vi "LVClass_Camera Set CameraSet.vi"(0 "Camera in":refnum<class "Camera.lvclass">, 5 "CameraSet":refnum<class "CameraSet.lvclass">, 7 "load_and_apply_connection_params":bool, 9 "load_and_apply_params":bool, 11 "error in (no error)":errorcluster) -> (4 "Camera out":refnum<class "Camera.lvclass">, 15 "error out":errorcluster)   [LabVIEW 2020, in "Camera.lvclass"]
doc: "Load and apply camera parameters from a CameraSet object.\n\n<B>CameraIn</B> : Camera object.\n<B>CameraOut</B> : Camera object.\n<B>CameraSet</B> : CameraSet object.\n<B>load_and_apply_connection_params</B> : try to load and apply connection parameters if true\n<B>load_and_apply_params</B> : try to load and apply parameters if true."
uses:
  Camera.lvclass
  CameraSet.lvclass
  Camera.lvclass/Camera.ctl
  LVClass_CameraSet Read CameraSet.vi
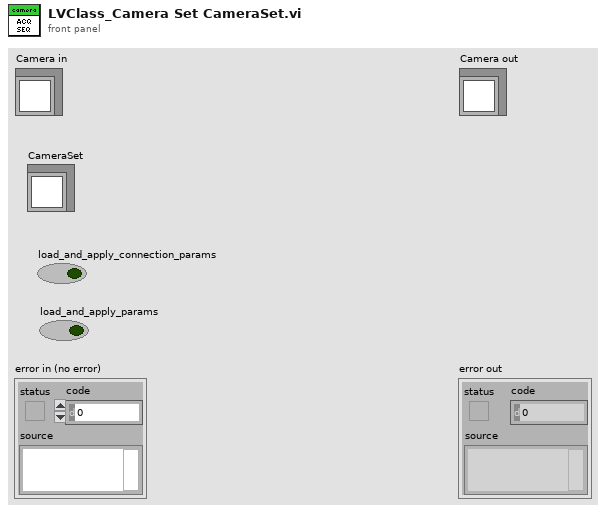
[diagram p1: front panel]
types:
  T1 = typedef "ClassID.ctl" = i64
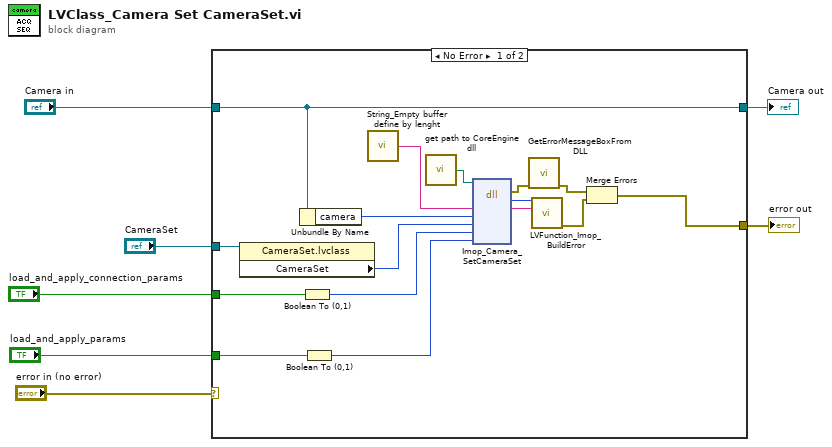
[diagram p0: block diagram]
diagram:
  n1 = case shown="No Error" "error in (no error)" {
    selector: "error in (no error)" -> [_ w25]
    tunnel: [w22 w25] -> w6
    tunnel: [w21 w24] -> w4
    tunnel: "Camera in" -> [w21 w24]
    tunnel: "CameraSet" -> [w13 _]
    tunnel: "load_and_apply_connection_params" -> [w12 _]
    tunnel: "load_and_apply_params" -> [w11 _]
    frame No Error {
      n2 = property class="CameraSet.lvclass"(reference=w13) -> ("CameraSet"=w8:T1)  [unwired: 1 in, 2 out]
      n3 = Unbundle By Name(w21) -> ("camera"=w20:T1)
      n4 = Boolean To (0,1)(Boolean=w12) -> (0, 1=w9:i16)
      n5 = Boolean To (0,1)(Boolean=w11) -> (0, 1=w10:i16)
      n6 = call "String_Empty buffer define by lenght.vi"() -> ("Empty buffer"=w23:string)  [unwired: 1 in]
      n7 = call "get path to CoreEngine dll.vi"() -> ("path to wavekit library"=w17:path)  [unwired: 14 in, 1 out]
      n8 = dll-call lib="D:/soft/HASO_v3/SVN_trunk/ImOpCoreEngine4_LV2011/DLLs/c_interface_vc100.dll" fn="Imop_Camera_SetCameraSet"(path in=w17, "message"=w23, "camera"=w20, "CameraSet"=w8, "load_and_apply_connection_params"=w9, "load_and_apply_params"=w10) -> (error out=w16:errorcluster, "return type"=w18:i32, "message"=w19:string)  [unwired: 6 in, 1 out]
      n9 = call "GetErrorMessageBoxFromDLL.vi"("error IN"=w16) -> ("error OUT"=w15:errorcluster)  [unwired: 10 in]
      n10 = call "LVFunction_Imop_BuildError.vi"("code"=w18, "String to Prepend to source (\"\")"=w19) -> ("error out"=w14:errorcluster)  [unwired: 13 in]
      n11 = Merge Errors(w15, w14) -> (w22:errorcluster)
    }
    frame Error {
    }
  }
  "error out" <- w6
  "Camera out" <- w4
